vi "generate file error.vi"(4 "message":string, 5 "call chain?":bool, 6 "source":string, 7 "severity":T1=enum."operation failed", 8 "exception in":T2 {"code" format="%.0x"}, 10 "file path":path, 11 "file error":T4) -> (0 "exception":T2 {"code" format="%.0x"})   [LabVIEW 2013, in "file errors.lvlib"]
uses:
  files/file errors.lvlib
  exception.lvlib
  context.ctl
  exception.ctl
  Variant Repository/Write Variant Repository/Write Exception Property.xnode
  <vilib>/Utility/VariantDataType/GetTypeInfo.vi
  <vilib>/Utility/VariantDataType/VariantType.lvlib
  files/file error.ctl
  severity.ctl
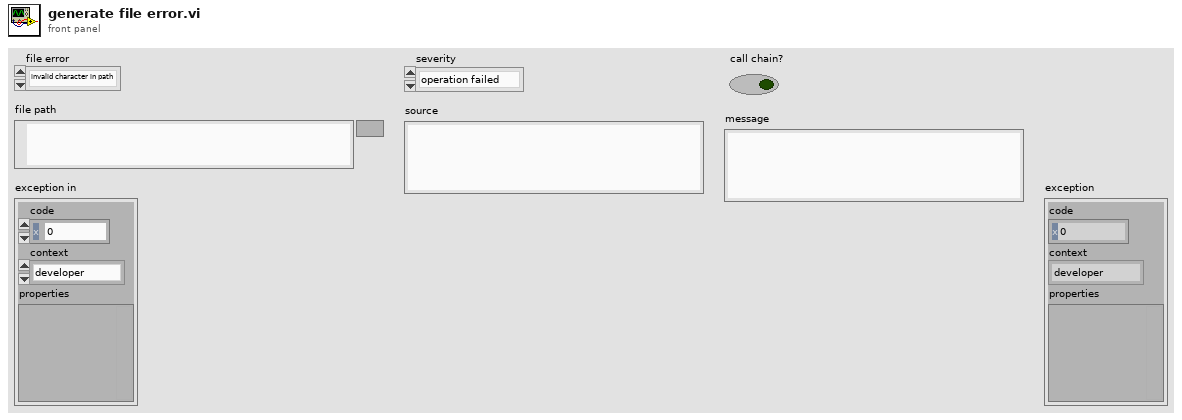
[diagram p1: front panel]
types:
  T1 = typedef "exception.lvlib/severity.ctl" = enum8{"unspecified", "operation failed", "data corruption", "system corruption", "critical unknown state"}
  T2 = typedef "exception.lvlib/exception.ctl" = cluster{"code":i32, "context":T3, "properties":variant}
  T3 = typedef "exception.lvlib/context.ctl" = enum16{"developer", "user interface", "standard", "limited", "deterministic"}
  T4 = typedef "file errors.lvlib/file error.ctl" = enum16{"invalid character in path"}
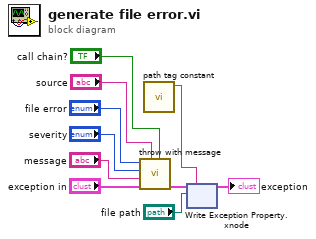
[diagram p0: block diagram]
diagram:
  n1 = call "throw with message.vi"("call chain?"="call chain?", "source"="source", "exception in"="exception in", "message"="message", "severity"="severity", "code"="file error") -> ("exception out"=w4:T2)  [unwired: 5 in]
  n2 = call "path tag constant.vi"() -> ("Tag"=w1:string)  [unwired: 11 in]
  n3 = xnode "Write Exception Property.xnode"("exception in"=w4, "Tag"=w1, "Value"="file path") -> ("exception out"=→"exception":T2)  [unwired: 1 out]
